vi "Teleop.vi"(10 "Match Info":T1={"Autonomous Elapsed Seconds"=0.0, "TeleOp Elapsed Seconds"=0.0, "Disabled Elapsed Seconds"=0.0, "Visited Autonomous"=FALSE, "Visited TeleOp"=FALSE, "Visited Disabled"=FALSE, "Autonomous Settings"={"Autonomous Style"=enum."Independent", "VI Refnum"=refnum}}, 11 "Call Context":T2) -> ()   [LabVIEW 2016]
doc: "This VI is called for each TeleOp packet received from the DS where the robot is not disabled. It is often used to read from the joysticks and update I/O or to update setpoints for timed control loops. It should complete and return within 20 milliseconds or it may miss DS packets."
uses:
  <vilib>/Rock Robotics/WPI/DriverStation/WPI_DriverStationDerivedRobotMode.ctl
  <vilib>/Rock Robotics/WPI/DriverStation/WPI_DriverStationMatch Info.ctl
  <vilib>/Rock Robotics/WPI/ThirdParty/CanMotor/TalonSRX/WPI_CANTalonSRX_APIFeedbackSelect.ctl
  <vilib>/Rock Robotics/WPI/ThirdParty/CanMotor/TalonSRX/WPI_CANTalonSRX_APIControlMode.ctl
  <vilib>/Rock Robotics/WPI/Utilities/WPI_GetSetVariantRefNum.vi
  <vilib>/Rock Robotics/Network Tables/NT Write Boolean Array.vi
  <vilib>/Rock Robotics/Network Tables/NT Write Numeric Array.vi
  <vilib>/Rock Robotics/Network Tables/NT Write Boolean.vi
  <vilib>/Rock Robotics/Network Tables/NT Read Boolean.vi
  <vilib>/Rock Robotics/Network Tables/NT Read Number.vi
panel:
  in  "F MM":dbl
  in  "D MM":dbl
  in  "I MM":dbl
  in  "P MM":dbl
  in  "F P":dbl
  in  "D P":dbl
  in  "I P":dbl
  in  "P P":dbl
  in  "F V":dbl
  in  "D V":dbl
  in  "I V":dbl
  in  "P V":dbl
  in  "Change Motor":bool
  out "Applied Throttle":dbl
  out "Sensor Position":dbl
  out "Sensor Velocity":dbl
  in  "Zero Position":bool
  out "Sensor Velocity":dbl(graph)
  out "Sensor Position":dbl(graph)
  out "Applied Throttle":dbl(graph)
  in  "Motion Magic Target Position":dbl format="%#_13g"
  in  "Max Acceleration":dbl format="%#_13g"
  in  "Cruise Velocity":dbl format="%#_13g"
  in  "Target Position":dbl format="%#_13g"
  in  "Motion Magic":bool
  in  "Position Loop":bool
  in  "Target Velocity":dbl format="%#_13g"
  in  "Velocity Loop":bool
  out "Sample Slider 0":dbl(slide) scale=0.0..5.0
  out "Sample Boolean 1":bool
  out "Sample Boolean 0":bool
  # "On = Right Motor\nOff = Left Motor"
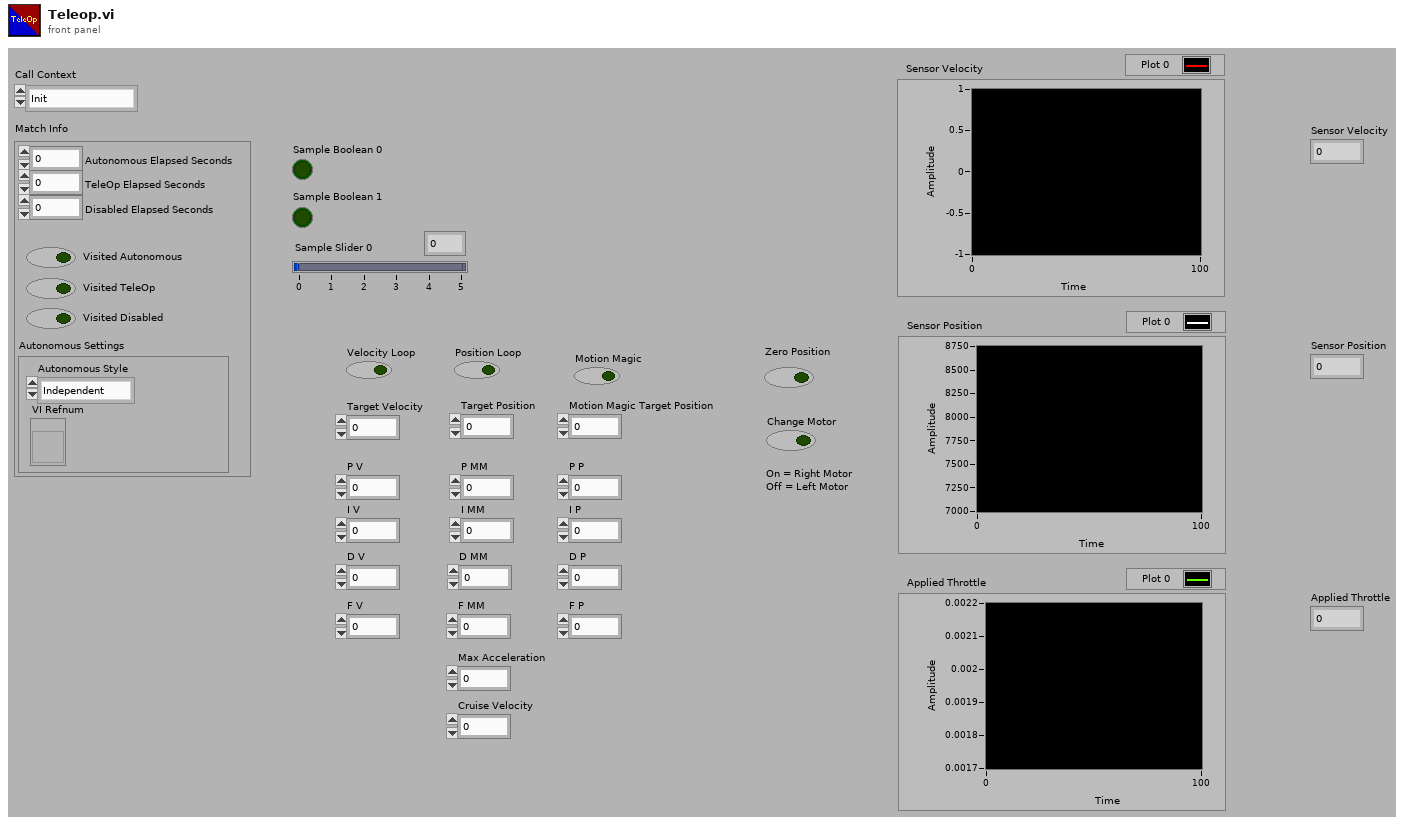
[diagram p1: front panel]
types:
  T1 = typedef "WPI_DriverStationMatch Info.ctl" = cluster{"Autonomous Elapsed Seconds":dbl, "TeleOp Elapsed Seconds":dbl, "Disabled Elapsed Seconds":dbl, "Visited Autonomous":bool, "Visited TeleOp":bool, "Visited Disabled":bool, "Autonomous Settings":cluster{"Autonomous Style":enum16{"Iterative", "Independent"}, "VI Refnum":refnum<vi>}}
  T2 = typedef "WPI_DriverStationDerivedRobotMode.ctl" = enum16{"Init", "Execute", "Stop"}
  T3 = typedef "WPI_CANTalonSRX_APIFeedbackSelect.ctl" = enum16{"Digital Quadrature Encoder", "Analog Potentiometer", "Analog Encoder", "Count on Quad-A (Rising-Edge)", "Count on Quad-A (Falling-Edge)", "CTR Magnetic Enc (Absolute)", "CTR Magnetic Enc (Relative)", "Pulse Width"}
  T4 = typedef "WPI_JoystickDevRef.ctl" = cluster{"Device":T5}
  T5 = typedef "WPI_JoystickDeviceEnum.ctl" = enum16{"USB 0", "USB 1", "USB 2", "USB 3", "USB 4", "USB 5"}
  T6 = typedef "WPI_MotorControlDeviceRef.ctl" = cluster{"DeviceStatus":errorcluster, "Type":T7, "PWM":cluster{"PWM Channel":T8, "DeadBand":T9}, "CAN":cluster{"Device Number":u8, "SetOutput VI Ref":variant, "GetOutput VI Ref":variant, "Enable VI Ref":variant, "Disable VI Ref":variant, "Data":variant}, "Invert":bool}
  T7 = typedef "WPI_MotorControlType.ctl" = enum16{"PWM", "CAN"}
  T8 = typedef "FPGA_DIOPWMChannel.ctl" = enum8{"PWM 0", "PWM 1", "PWM 2", "PWM 3", "PWM 4", "PWM 5", "PWM 6", "PWM 7", "PWM 8", "PWM 9", "PWM MXP 0", "PWM MXP 1", "PWM MXP 2", "PWM MXP 3", "PWM MXP 4", "PWM MXP 5", "PWM MXP 6", "PWM MXP 7", "PWM MXP 8", "PWM MXP 9", "Invalid"}
  T9 = typedef "WPI_PWMDeadband.ctl" = cluster{"Name":string, "maxPositivePwm":i32, "minPositivePwm":i32, "centerPwm":i32, "maxNegativePwm":i32, "minNegativePwm":i32, "angularRange":u16}
  T10 = cluster{"Velocity Loop":bool, "Position Loop":bool, "Motion Magic":bool}
  T11 = typedef "WPI_CANTalonSRX_GlobalStatus.ctl" = cluster{"Applied Throttle":dbl, "Module Enabled":bool, "CAN Error":errorcluster, "Closed Loop Error":dbl, "Forward Limit Switch Closed":bool, "Reverse Limit Switch Closed":bool, "Sensor Position":dbl, "Sensor Velocity":dbl, "Current":dbl, "Sticky Fault - Over Temp":bool, "Sticky Fault - Under Voltage":bool, "Sticky Fault - Forward Limit":bool, "Sticky Fault - Reverse Limit":bool, "Sticky Fault - Forward Soft Limit":bool, "Sticky Fault - Reverse Soft Limit":bool, "Brake is Enabled":bool, "Encoder Position":dbl, "Encoder Velocity":dbl, "Encoder Index Count":dbl, "Encoder A Pin State":bool, "Encoder B Pin State":bool, "Encoder Index Pin State":bool, "Analog In":dbl, "Analog In Velocity":dbl, "Temperature (C)":dbl, "Battery Voltage":dbl, "Control 5 Is Supported":bool, "Current Profile Slot Select":dbl, "Pos Div 8":bool, "Vel Div 4":bool, "Pulse Width Position":i32, "Pulse Width Velocity":i32, "Pulse Width Rise To Rise (us)":i32, "Pulse Width Rise To Fall (us)":i32, "Mot Prof Active Is Under Run":bool, "Mot Prof Active Has Under Run":bool, "Mot Prof Active Is Last":bool, "Mot Prof Active Velocity Only":bool, "Mot Prof Active Is Valid":bool, "Mot Prof Buffer Is Full":bool, "Mot Prof Active Profile Slot Select":i32, "Mot Prof NextID":i32, "Mot Prof Count":i32, "Mot Prof Active Velocity":dbl, "Mot Prof Active Position":dbl, "Mot Prof Output Enable":i32, "UsageFrame":u32, "Motion Magic Active Trajectory":cluster{"Velocity":dbl, "Position":dbl}}
  T12 = typedef "WPI_CANTalonSRX_APIControlMode.ctl" = enum8{"Percent VBus", "Speed", "Position", "Slave", "Unchanged / Invalid", "Voltage Compensation", "Current", "Motion Profile", "Motion Magic"}
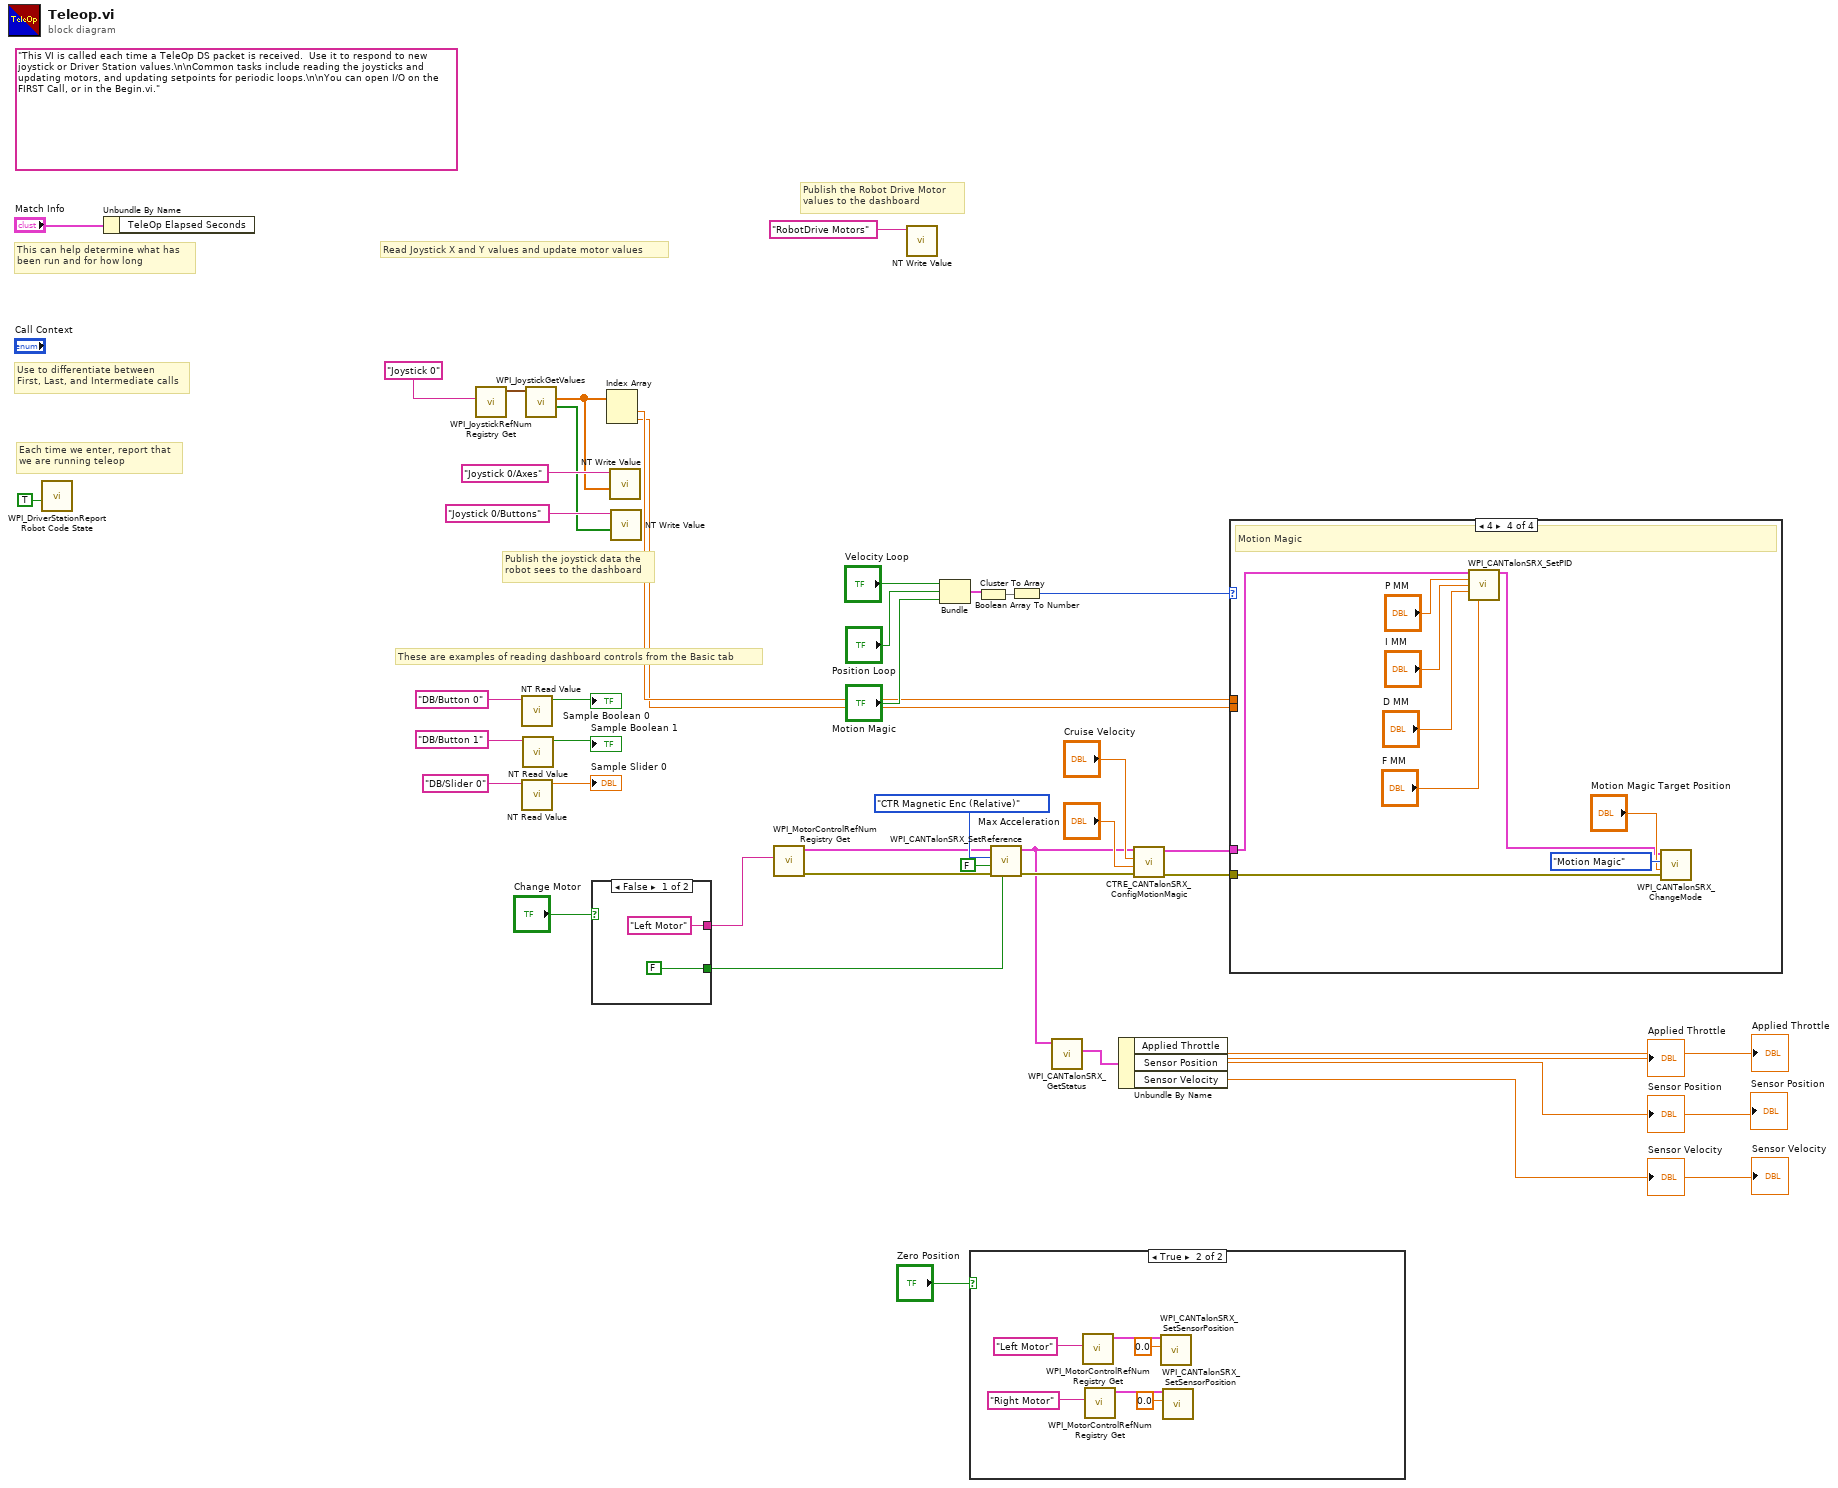
[diagram p0: block diagram]
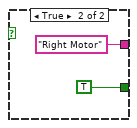
[diagram p2: hidden frame]
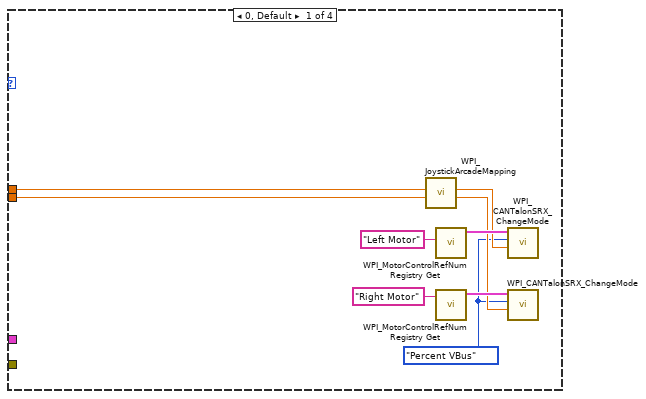
[diagram p4: hidden frame]
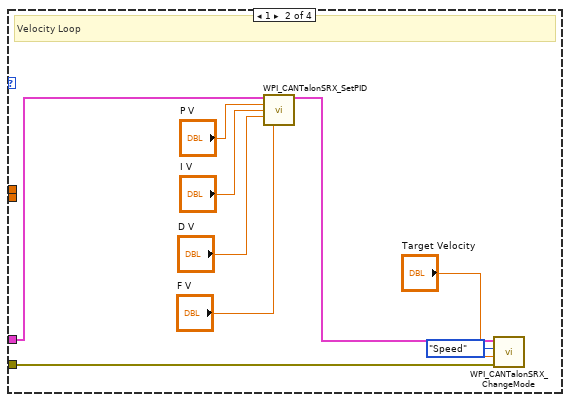
[diagram p5: hidden frame]
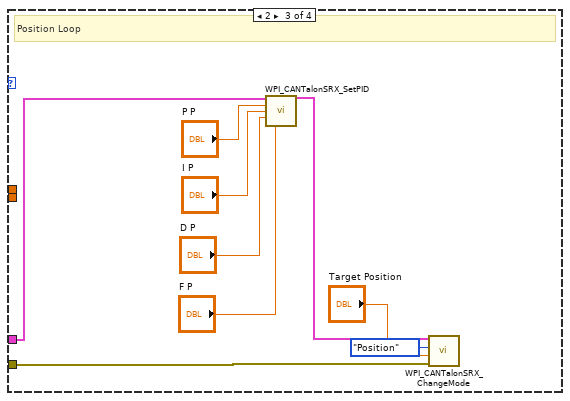
[diagram p6: hidden frame]
diagram:
  (unwired) "This VI is called each time a TeleOp DS packet is received.  Use it to respond to new joystick or Driver Station values.\n\nCommon tasks include reading the joysticks and updating motors, and updating setpoints for periodic loops.\n\nYou can open I/O on the FIRST Call, or in the Begin.vi."
  # "These are examples of reading dashboard controls from the Basic tab"
  # "Publish the Robot Drive Motor\nvalues to the dashboard"
  # "Publish the joystick data the\nrobot sees to the dashboard"
  # "Each time we enter, report that\nwe are running teleop"
  # "Use to differentiate between\nFirst, Last, and Intermediate calls"
  # "This can help determine what has\nbeen run and for how long"
  # "Read Joystick X and Y values and update motor values"
  n1 = call <vilib>:"WPI_DriverStationReport Robot Code State.vi"("TeleOp"=TRUE ("Autonomous")) -> ()  [unwired: 10 in, 1 out]
  n2 = Unbundle By Name("Match Info") -> ()  [unwired: 1 out]
  n3 = call <vilib>:"WPI_JoystickRefNum Registry Get.vi"("refnum name"="Joystick 0") -> ("JoystickDevRef"=w39:T4)  [unwired: 1 in, 9 out]
  n4 = call-poly <vilib>:"NT Read Value.vi"("Name"="DB/Button 0" ("refnum name")) -> ("Boolean"=→"Sample Boolean 0":bool)  [unwired: 9 in, 1 out]
  n5 = call-poly <vilib>:"NT Read Value.vi"("Name"="DB/Slider 0" ("refnum name")) -> ("Numeric"=→"Sample Slider 0":dbl)  [unwired: 9 in, 1 out]
  n6 = call-poly <vilib>:"NT Read Value.vi"("Name"="DB/Button 1" ("refnum name")) -> ("Boolean"=→"Sample Boolean 1":bool)  [unwired: 9 in, 1 out]
  n7 = call <vilib>:"WPI_JoystickGetValues.vi"("JoystickDevRef"=w39) -> ("Buttons"=w34:bool[], "Axes"=w35:dbl[])  [unwired: 6 in, 3 out]
  n8 = case shown="False" "Change Motor" {
    tunnel: ["Left Motor" ("refnum name") "Right Motor" ("refnum name")] -> w2
    tunnel: [FALSE ("Reverse Closed-Loop Output") TRUE ("Reverse Closed-Loop Output")] -> w1
    frame False {
    }
    frame True {
    }
  }
  n9 = Index Array(array=w35) -> (element #1=w12:dbl, element #2=w11:dbl)  [unwired: 2 in]
  n10 = call-poly <vilib>:"NT Write Value.vi"("Numeric Array"=w35, "Name"="Joystick 0/Axes") -> ()  [unwired: 9 in, 1 out]
  n11 = call-poly <vilib>:"NT Write Value.vi"("Boolean Array"=w34, "Name"="Joystick 0/Buttons") -> ()  [unwired: 9 in, 1 out]
  n12 = call <vilib>:"WPI_MotorControlRefNum Registry Get.vi"("refnum name"=w2) -> ("error out"=w15:errorcluster, "MotorControlDevRef"=w24:T6)  [unwired: 9 in]
  n13 = call-poly <vilib>:"NT Write Value.vi"("Name"="RobotDrive Motors") -> ()  [unwired: 10 in, 1 out]
  n14 = Bundle("Velocity Loop"="Velocity Loop", "Position Loop"="Position Loop", "Motion Magic"="Motion Magic") -> (w8:T10)  [unwired: 1 in]
  n15 = case shown="True" "Zero Position" {
    frame False {
    }
    frame True {
      n16 = call <vilib>:"WPI_MotorControlRefNum Registry Get.vi"("refnum name"="Left Motor") -> ("MotorControlDevRef"=w51:T6)  [unwired: 9 in, 1 out]
      n17 = call <vilib>:"WPI_MotorControlRefNum Registry Get.vi"("refnum name"="Right Motor") -> ("MotorControlDevRef"=w48:T6)  [unwired: 9 in, 1 out]
      n18 = call <vilib>:"WPI_CANTalonSRX_SetSensorPosition.vi"("New Sensor Position"=0.0, "CAN Talon SRX Ref"=w51) -> ()  [unwired: 8 in, 2 out]
      n19 = call <vilib>:"WPI_CANTalonSRX_SetSensorPosition.vi"("New Sensor Position"=0.0, "CAN Talon SRX Ref"=w48) -> ()  [unwired: 8 in, 2 out]
    }
  }
  n20 = Cluster To Array(cluster=w8) -> (array=w23:bool[])
  n21 = call <vilib>:"WPI_CANTalonSRX_SetReference.vi"("Reverse Closed-Loop Output"=w1, "error in (no error)"=w15, "Reverse Feedback Sensor"=FALSE, "Feedback Reference"=WPI_CANTalonSRX_APIFeedbackSelect."CTR Magnetic Enc (Relative)", "CAN Talon SRX Ref"=w24) -> ("error out"=w14:errorcluster, "CAN Talon SRX Ref"=w10:T6)  [unwired: 5 in]
  n22 = Boolean Array To Number(Boolean array=w23) -> (number=w22:u32)
  n23 = call <vilib>:"WPI_CANTalonSRX_GetStatus.vi"("CAN Talon SRX Ref"=w10) -> ("Talon SRX Status"=w9:T11)  [unwired: 8 in, 2 out]
  n24 = Unbundle By Name(w9) -> ("Applied Throttle"=→"Applied Throttle" →"Applied Throttle":dbl, "Sensor Position"=→"Sensor Position" →"Sensor Position":dbl, "Sensor Velocity"=→"Sensor Velocity" →"Sensor Velocity":dbl)
  n25 = call <vilib>:"CTRE_CANTalonSRX_ConfigMotionMagic.vi"("error in (no error)"=w14, "Max Acceleration"="Max Acceleration", "Cruise Velocity"="Cruise Velocity", "CAN Talon SRX Ref"=w10) -> ("error out"=w13:errorcluster, "CAN Talon SRX Ref Out"=w18:T6)  [unwired: 6 in]
  n26 = case shown="4" w22 {
    tunnel: w18 -> [_ w62 w71 w80]
    tunnel: w13 -> [_ w68 w76 w87]
    tunnel: w12 -> [w56 _ _ _]
    tunnel: w11 -> [w55 _ _ _]
    frame 0, Default {
      w52 = WPI_CANTalonSRX_APIControlMode."Percent VBus" ("Control Mode")
      n27 = call <vilib>:"WPI_JoystickArcadeMapping.vi"("Y axis value"=w55, "X axis value"=w56) -> ("Right Motor Value"=w53:dbl, "Left Motor Value"=w54:dbl)  [unwired: 8 in]
      n28 = call <vilib>:"WPI_MotorControlRefNum Registry Get.vi"("refnum name"="Left Motor") -> ("MotorControlDevRef"=w58:T6)  [unwired: 9 in, 1 out]
      n29 = call <vilib>:"WPI_MotorControlRefNum Registry Get.vi"("refnum name"="Right Motor") -> ("MotorControlDevRef"=w57:T6)  [unwired: 9 in, 1 out]
      n30 = call <vilib>:"WPI_CANTalonSRX_ChangeMode.vi"("Output"=w54, "Control Mode"=w52, "CAN Talon SRX Ref"=w58) -> ()  [unwired: 7 in, 2 out]
      n31 = call <vilib>:"WPI_CANTalonSRX_ChangeMode.vi"("Output"=w53, "Control Mode"=w52, "CAN Talon SRX Ref"=w57) -> ()  [unwired: 7 in, 2 out]
    }
    frame 1 {
      # "Velocity Loop"
      n32 = call <vilib>:"WPI_CANTalonSRX_SetPID.vi"("CAN Talon SRX Ref"=w62, "P"="P V", "I"="I V", "D"="D V", "F"="F V") -> ("CAN Talon SRX Ref"=w61:T6)  [unwired: 9 in, 1 out]
      n33 = call <vilib>:"WPI_CANTalonSRX_ChangeMode.vi"("error in (no error)"=w68, "Output"="Target Velocity", "Control Mode"=WPI_CANTalonSRX_APIControlMode."Speed", "CAN Talon SRX Ref"=w61) -> ()  [unwired: 6 in, 2 out]
    }
    frame 2 {
      # "Position Loop"
      n34 = call <vilib>:"WPI_CANTalonSRX_SetPID.vi"("CAN Talon SRX Ref"=w71, "P"="P P", "I"="I P", "D"="D P", "F"="F P") -> ("CAN Talon SRX Ref"=w70:T6)  [unwired: 9 in, 1 out]
      n35 = call <vilib>:"WPI_CANTalonSRX_ChangeMode.vi"("error in (no error)"=w76, "Output"="Target Position", "Control Mode"=WPI_CANTalonSRX_APIControlMode."Position", "CAN Talon SRX Ref"=w70) -> ()  [unwired: 6 in, 2 out]
    }
    frame 4 {
      # "Motion Magic"
      n36 = call <vilib>:"WPI_CANTalonSRX_SetPID.vi"("CAN Talon SRX Ref"=w80, "P"="P MM", "I"="I MM", "D"="D MM", "F"="F MM") -> ("CAN Talon SRX Ref"=w79:T6)  [unwired: 9 in, 1 out]
      n37 = call <vilib>:"WPI_CANTalonSRX_ChangeMode.vi"("error in (no error)"=w87, "Output"="Motion Magic Target Position", "Control Mode"=WPI_CANTalonSRX_APIControlMode."Motion Magic", "CAN Talon SRX Ref"=w79) -> ()  [unwired: 6 in, 2 out]
    }
  }
